vi "FT_Set_Deadman_Timeout.vi"() -> ()   [LabVIEW 2019, in "D2XX_Functions.lvlib"]
uses:
  D2XX_Functions.lvlib
  CDM v2.12.36.4 WHQL Certified/i386/ftd2xx.dll
panel:
  out "FT_Status":u32(ring) items=["FT_OK", "FT_INVALID_HANDLE", "FT_DEVICE_NOT_FOUND", "FT_DEVICE_NOT_OPENED", "FT_IO_ERROR", "FT_INSUFFICIENT_RESOURCES", "FT_INVALID_PARAMETER", "FT_INVALID_BAUD_RATE", "FT_DEVICE_NOT_OPENED_FOR_ERASE", "FT_DEVICE_NOT_OPENED_FOR_WRITE", "FT_FAILED_TO_WRITE_DEVICE", "FT_EEPROM_READ_FAILED", "FT_EEPROM_WRITE_FAILED", "FT_EEPROM_ERASE_FAILED", "FT_EEPROM_NOT_PRESENT", "FT_EEPROM_NOT_PROGRAMMED", "FT_INVALID_ARGS", "FT_NOT_SUPPORTED", "FT_OTHER_ERROR"]
  in  "DeadmanTimeout":u32=5000
  in  "Handle":u32
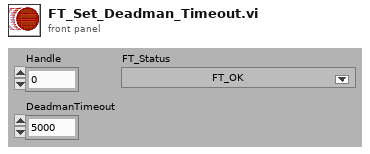
[diagram p1: front panel]
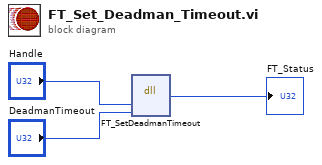
[diagram p0: block diagram]
diagram:
  n1 = dll-call lib="C:/Users/patrick/Documents/GitHub/Relay-Box/lvsrc/CDM v2.12.36.4 WHQL Certified/i386/FTD2XX.dll" fn="FT_SetDeadmanTimeout"("Handle"="Handle", "DeadmanTimeout"="DeadmanTimeout") -> ("FT_Status"=→"FT_Status":u32)  [unwired: 5 in, 2 out]
